vi "Shooter Teleop.vi"(10 "LimeLightDistance?":bool, 11 "Setpoint":dbl) -> ()   [LabVIEW 2019]
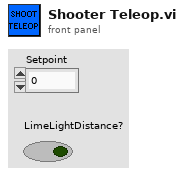
[diagram p1: front panel]
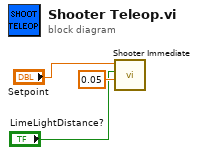
[diagram p0: block diagram]
diagram:
  n1 = call "Shooter Immediate.vi"("Deadband Value"=0.05, "LimeLightDistance?"="LimeLightDistance?", "Setpoint"="Setpoint") -> ()  [unwired: 8 in, 1 out]
